vi "Main v0.2.vi"() -> ()   [LabVIEW 2017]
doc: "This template is for the Queued Message Handler design pattern.\n\nThe Event Handling Loop generates messages based on user interface actions.\n\nThe Message Handling Loop processes messages generated by the Event Handling Loop, or by other messages. The messages are string values, so new messages can be added easily to the Message Cases case structure in the Message Handling Loop. Each message cluster can also provide an optional value for Message Data, which is a variant that can be converted to whatever message-specific data is required."
uses:
  Controls/Main Tabs.ctl
  Controls/Auto.ctl
  RT/Controls/Auto Delays.ctl
  RT/Controls/Auto Times.ctl
  Controls/UI Data.ctl
  support/Message Queue/Enqueue Message (Single).vi
  <vilib>/Utility/error.llb/Error Cluster From Error Code.vi
  <vilib>/ErrorRing/Error Ring.xnode
  support/Message Queue/Message Queue.lvlib
  support/User Event - Stop/User Event - Stop.lvlib
panel:
  out "Date-Time":string caption="Dip-Tube Assembly Automation (HMI) v0.2"
  out "Main Tab":T1
  in  "Autocycle":T2
  in  "Manual":bool
  in  "Parameters":bool
  in  "Maintenance":bool
  in  "Save Para":bool
  in  "Home Para":bool
  in  "ParaTab":T3(tab)
  in  "StopperRearDelay":dbl format="%#.2f"
  in  "StopperFrontDelay":dbl format="%#.2f"
  in  "MaxAlarms":dbl caption="Max Alarms in 1 Minute" format="%#.2f"
  in  "MaxConsecutive":dbl caption="Max Consecutive Alarms" format="%#.2f"
  in  "Gate Close Delay":dbl format="%#.2f"
  in  "Gate Open Delay":dbl format="%#.2f"
  in  "BF Off Delay":dbl format="%#.2f"
  in  "BF On Delay":dbl format="%#.2f"
  in  "DelayAfterReject":dbl format="%#.2f"
  in  "MeasurementTime":dbl format="%#.2f"
  in  "DelayAfterMesFront":dbl format="%#.2f"
  in  "DelayAfterCut":dbl format="%#.2f"
  in  "DelayAfterCutClamp":dbl format="%#.2f"
  in  "DelayAfterInsClamp":dbl format="%#.2f"
  in  "DelayToClose":dbl format="%#.2f"
  in  "DelayToOpen":dbl format="%#.2f"
  in  "DelayAfterInsertion":dbl format="%#.2f"
  in  "DelayBeforeInsertion":dbl format="%#.2f"
  in  "AgitatorUpTime":dbl format="%#.2f"
  in  "AgitatorDownTime":dbl format="%#.2f"
  in  "Enable Index?":bool
  in  "Enable PF?":bool
  in  "Auto Delays":T4={"Agitator Delays"=[1000], "TF Delays"=[1000], "Insertion Delays"=[1000, 1000], "Cutting Delays"=[1000, 1000], "PF Delays"=[1000]}
  in  "Enable Cutting?":bool
  in  "Enable Insertion?":bool
  in  "Run Manual":bool
  in  "Enable TF?":bool
  in  "Home Manual":bool
  out "Status":T6
  in  "All IO":bool
  in  "Stats":bool
  in  "Home AC":bool
  out "Status":string
  out "Count":dbl format="%06.0f"
  out "Count 3":dbl caption="Cycle Time" format="%0.2f"
  out "Count 2":dbl caption="Rejects" format="%06.0f"
  in  "Statuses":string[][](table)
  in  "Exit":bool
  # "Vision Harmony Dip-Tube Assembly Automation"
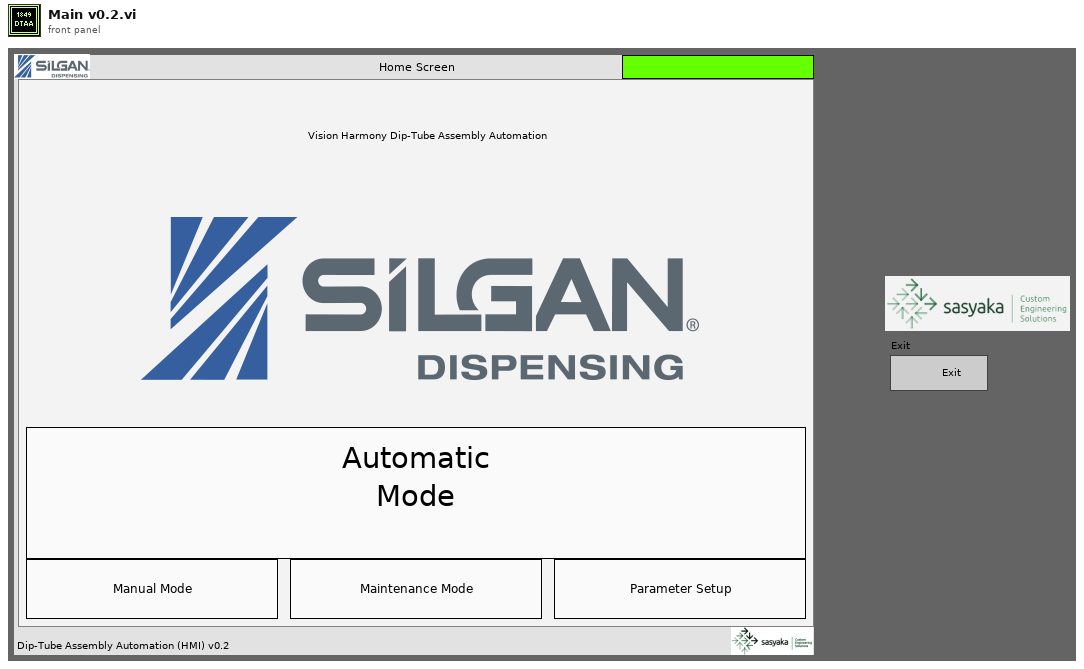
[diagram p1: front panel]
types:
  T1 = typedef "Main Tabs.ctl" = enum32{"Home Screen", "Parameter Setup", "Manual Mode", "Autocycle"}
  T2 = typedef "Auto.ctl" = bool
  T3 = enum32{"General & Indexing", "Bowl Feeder & Pump Conveyor", "Cutting, Measurement & Rejection", "Tube Feeder & Insertion"}
  T4 = typedef "Auto Delays.ctl" = cluster{"Agitator Delays":u32[], "TF Delays":u32[], "Insertion Delays":u32[], "Cutting Delays":u32[], "PF Delays":u32[]}
  T5 = typedef "Auto Times.ctl" = cluster{"Index Time":u32, "TF Time":u32, "Insertion Time":u32, "Cutting Time":u32, "PF Time":u32}
  T6 = cluster{"Auto Times":T5, "error out":errorcluster}
  T7 = typedef "UI Data.ctl" = cluster{"Main Tab":refnum<vi>}
  T8 = typedef "Message Queue.lvlib/All Message Queues.ctl" = cluster{"UI":refnum<queue>}
  T9 = enum8{"Enabled", "Disabled", "Disabled and Grayed Out"}
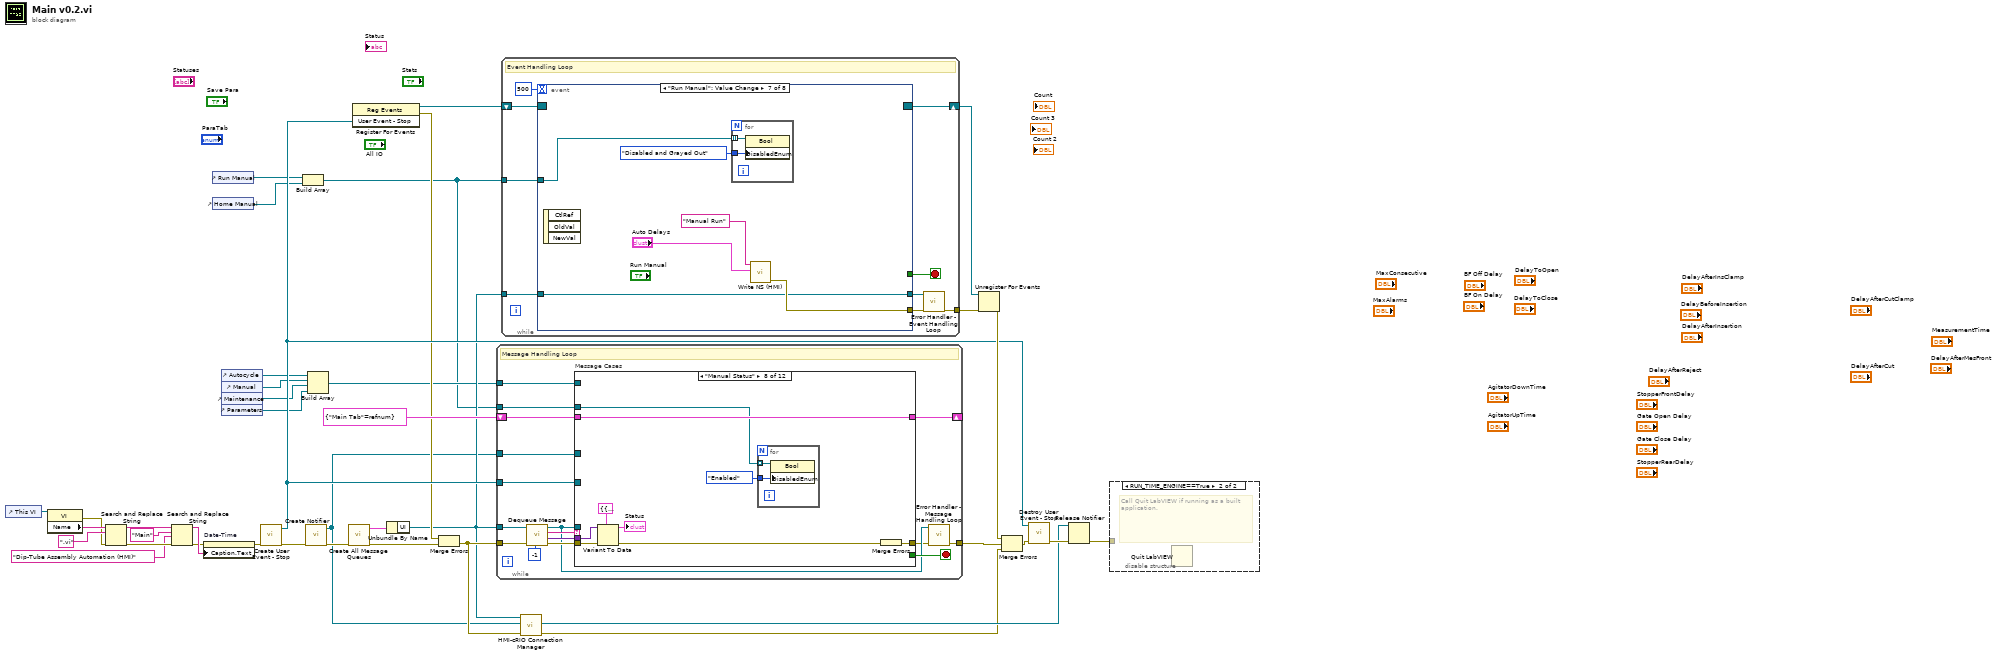
[diagram p0: block diagram]
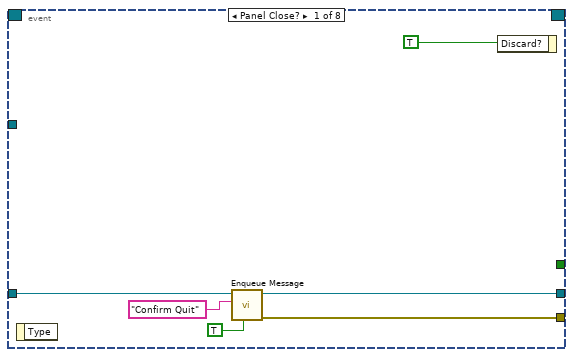
[diagram p2: hidden frame]
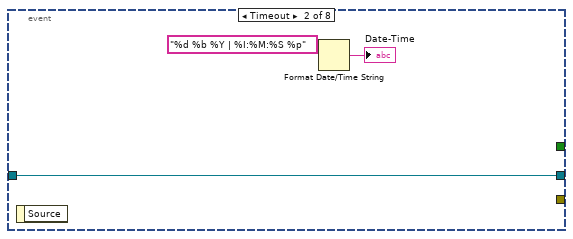
[diagram p3: hidden frame]
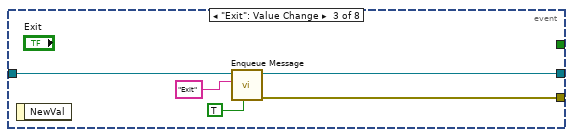
[diagram p4: hidden frame]
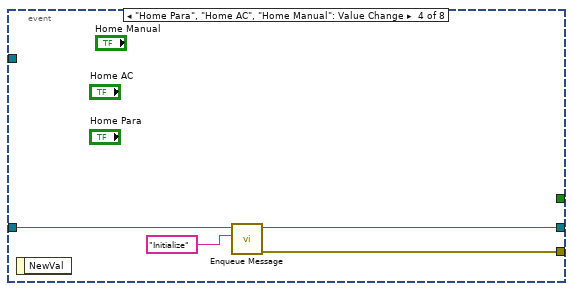
[diagram p5: hidden frame]
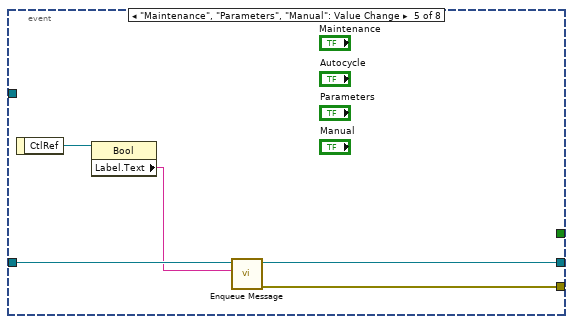
[diagram p6: hidden frame]
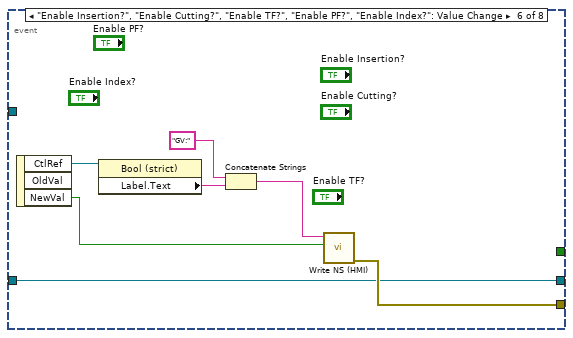
[diagram p7: hidden frame]
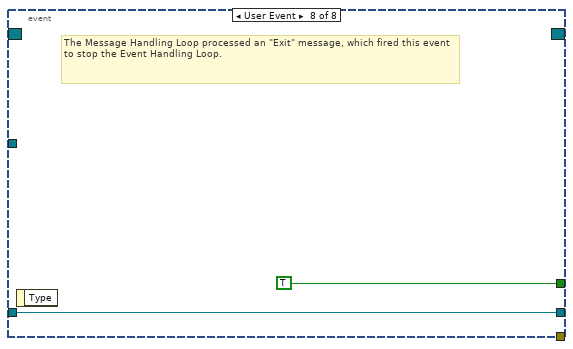
[diagram p8: hidden frame]
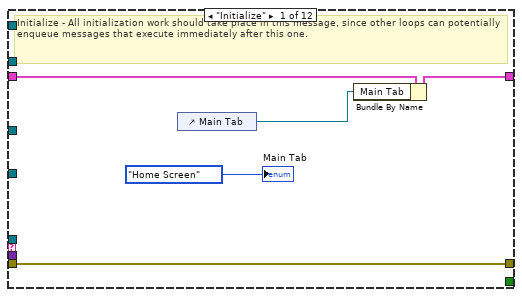
[diagram p9: hidden frame]
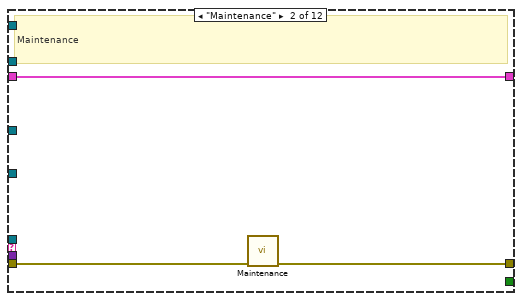
[diagram p10: hidden frame]
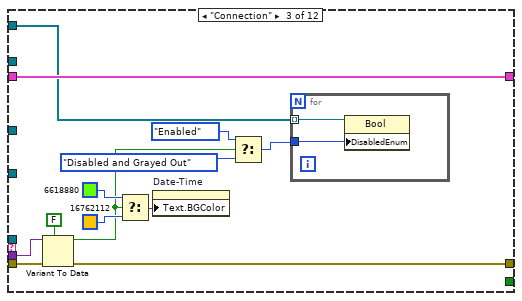
[diagram p11: hidden frame]
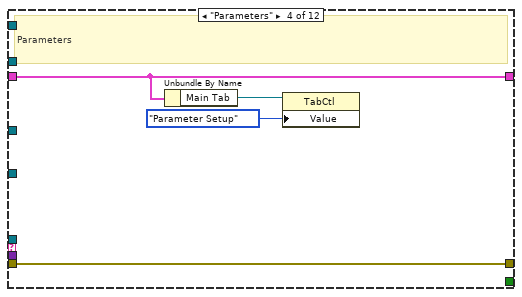
[diagram p12: hidden frame]
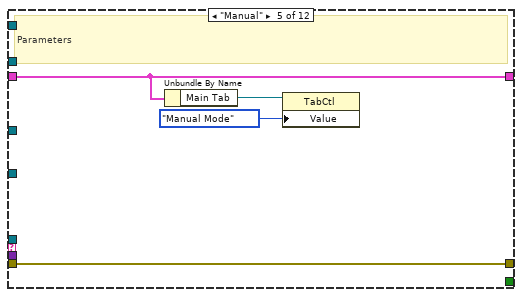
[diagram p13: hidden frame]
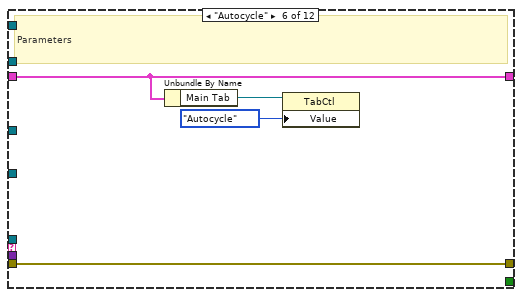
[diagram p14: hidden frame]
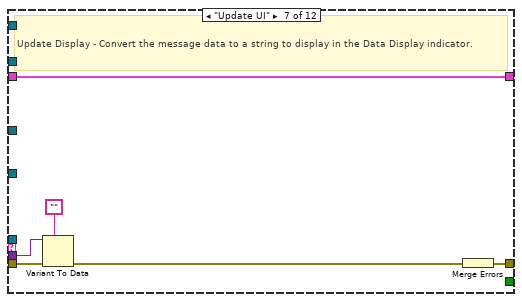
[diagram p15: hidden frame]
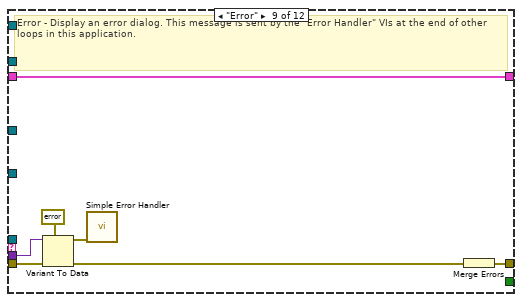
[diagram p16: hidden frame]
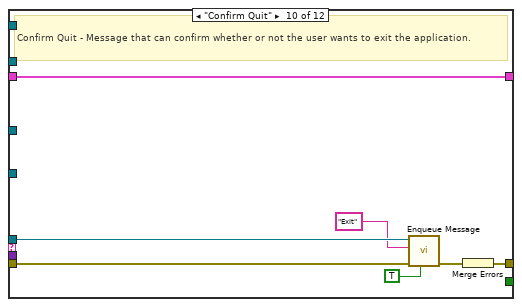
[diagram p17: hidden frame]
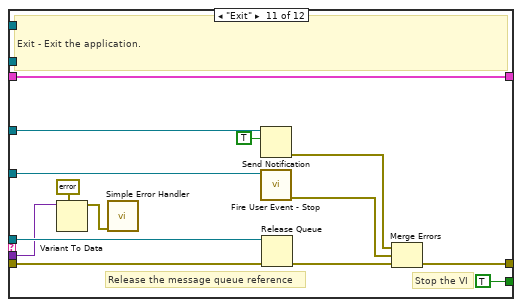
[diagram p18: hidden frame]
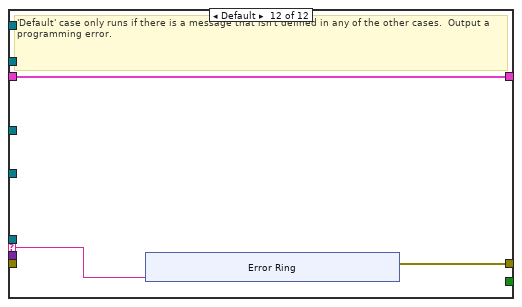
[diagram p19: hidden frame]
diagram:
  n1 = control-ref of="This VI"() -> (w8:refnum<vi>)
  n2 = property class="VI"(reference=w8) -> (error out=w7:errorcluster, "Name"=w14:string)  [unwired: 1 in, 1 out]
  n3 = Search and Replace String(input string=w14, search string=".vi", error in=w7) -> (result string=w12:string, error out=w11:errorcluster)  [unwired: 5 in, 2 out]
  n4 = Search and Replace String(input string=w12, search string="Main", replace string="Dip-Tube Assembly Automation (HMI)" ("replace string (\"\")"), error in=w11) -> (result string=w6:string, error out=w5:errorcluster)  [unwired: 4 in, 2 out]
  n5 = property on="Date-Time" class="Str"(error in=w5, "Caption.Text"=w6) -> (error out=w4:errorcluster)  [unwired: 1 in, 1 out]
  n6 = control-ref of="Run Manual"() -> (w3:refnum<vi>)
  n7 = control-ref of="Home Manual"() -> (w2:refnum<vi>)
  n8 = control-ref of="Autocycle"() -> (w19:refnum<vi>)
  n9 = control-ref of="Manual"() -> (w18:refnum<vi>)
  n10 = control-ref of="Maintenance"() -> (w17:refnum<vi>)
  n11 = control-ref of="Parameters"() -> (w16:refnum<vi>)
  n12 = call "Create User Event - Stop.vi"("error in (no error)"=w4) -> ("error out"=w26:errorcluster, "User Event - Stop"=w30:refnum<user-event>)  [unwired: 9 in]
  n13 = Build Array(w3, w2) -> (w1:refnum<vi>[])
  n14 = call "Create Notifier.vi"("error in (no error)"=w26) -> ("error out"=w25:errorcluster, "notifier out"=w20:refnum<notifier>)  [unwired: 9 in]
  n15 = Build Array(w19, w18, w17, w16) -> (w15:refnum<vi>[])
  n16 = call "Create All Message Queues.vi"("error in (no error)"=w25) -> ("error out"=w39:errorcluster, "Message Queues out"=w38:T8)  [unwired: 9 in]
  n17 = register-events(w30) -> (reference out=w31:refnum<event-registration>, error out=w29:errorcluster)  [unwired: 2 in]
  n18 = Unbundle By Name(w38) -> ("UI"=w27:refnum<queue>)
  n19 = Merge Errors(w29, w39) -> (w28:errorcluster)
  n20 = while {
    tunnel: w27 -> [w47]
    shift-right: [w54] -> _
    shift-left: T7 {"Main Tab"=refnum} ("Data Cluster") -> [w55]
    tunnel: w30 -> [w52]
    tunnel: w28 -> [w51]
    tunnel: [w45] -> w37
    tunnel: w20 -> [w42]
    tunnel: w15 -> [w41]
    tunnel: w1 -> [w40]
    stop <- w53 stop-if-true
    # "Message Handling Loop"
    n21 = call "Dequeue Message.vi"("timeout"=-1, "error in (no error)"=w51, "Message Queue"=w47) -> ("error out"=w50:errorcluster, "Message Data"=w48:variant, "Message"=w49:string, "dup Message Queue"=w46:refnum<queue>)  [unwired: 5 in]
    n22 = case "Message Cases" shown="\"Manual Status\"" w49 {
      selector: w49 -> [_ _ _ _ _ _ _ _ _ _ _ w136]
      tunnel: w46 -> [_ _ _ _ _ _ _ _ _ w117 w135 _]
      tunnel: w50 -> [w60 w62 w74 w82 w86 w90 w94 w103 w114 w121 w128 _]
      tunnel: [w60 w61 w73 w82 w86 w90 w95 w104 w108 w119 w131 w137] -> w44
      tunnel: w55 -> [w59 w63 w76 w81 w85 w89 w96 w105 w113 w120 w134 w138]
      tunnel: [w58 w63 w76 w81 w85 w89 w96 w105 w113 w120 w134 w138] -> w54
      tunnel: [_ _ _ _ _ _ _ _ _ _ TRUE _] -> w53
      tunnel: w48 -> [_ _ w72 _ _ _ w93 w102 w112 _ w125 _]
      tunnel: w52 -> [_ _ _ _ _ _ _ _ _ _ w130 _]
      tunnel: w42 -> [_ _ _ _ _ _ _ _ _ _ w124 _]
      tunnel: w41 -> [_ _ w68 _ _ _ _ _ _ _ _ _]
      tunnel: w40 -> [_ _ _ _ _ _ _ w97 _ _ _ _]
      frame "Initialize" {
        # "Initialize - All initialization work should take place in this message, since other loops can potentially enqueue messages that execute immediately after this one."
        n23 = control-ref of="Main Tab"() -> (w57:refnum<vi>)
        n24 = Bundle By Name(cluster=w59, "Main Tab"=w57) -> (w58:T7)
        "Main Tab" <- Main_Tabs."Home Screen" ("Main Tab")
      }
      frame "Maintenance" {
        # "Maintenance"
        n25 = call "Maintenance.vi"("Error In"=w62) -> ("Error out"=w61:errorcluster)  [unwired: 10 in]
      }
      frame "Connection" {
        n26 = Variant To Data(error in=w74, type=FALSE, Variant=w72) -> (data=w67:bool, error out=w73:errorcluster)
        n27 = Select(t=u32 6618880 ("Text.Text Colors:BG Color"), s=w67, f=u32 16762112 ("Text.Text Colors:BG Color")) -> (s? t:f=w69:u32)
        n28 = property on="Date-Time" class="Str"("Text.BGColor"=w69) -> ()  [unwired: 2 in, 2 out]
        n29 = Select(t=T9."Enabled" ("Disabled"), s=w67, f=T9."Disabled and Grayed Out") -> (s? t:f=w65:T9)
        n30 = for {
          tunnel: w68 -> [w78] mode=indexing
          tunnel: w65 -> [w77]
          n31 = property class="Bool"(reference=w78, "DisabledEnum"=w77) -> ()  [unwired: 1 in, 2 out]
        }
      }
      frame "Parameters" {
        # "Parameters"
        n32 = Unbundle By Name(w81) -> ("Main Tab"=w80:refnum<vi>)
        n33 = property class="TabCtl"(reference=w80, "Value"=Main_Tabs."Parameter Setup" ("Main Tab")) -> ()  [unwired: 1 in, 2 out]
      }
      frame "Manual" {
        # "Parameters"
        n34 = Unbundle By Name(w85) -> ("Main Tab"=w84:refnum<vi>)
        n35 = property class="TabCtl"(reference=w84, "Value"=Main_Tabs."Manual Mode" ("Main Tab")) -> ()  [unwired: 1 in, 2 out]
      }
      frame "Autocycle" {
        # "Parameters"
        n36 = Unbundle By Name(w89) -> ("Main Tab"=w88:refnum<vi>)
        n37 = property class="TabCtl"(reference=w88, "Value"=Main_Tabs."Autocycle" ("Main Tab")) -> ()  [unwired: 1 in, 2 out]
      }
      frame "Update UI" {
        # "Update Display - Convert the message data to a string to display in the Data Display indicator."
        n38 = Variant To Data(error in=w94, type="", Variant=w93) -> (error out=w91:errorcluster)  [unwired: 1 out]
        n39 = Merge Errors(w91) -> (w95:errorcluster)
      }
      frame "Manual Status" {
        n40 = Variant To Data(error in=w103, type=T6 {"Auto Times"={"Index Time"=0, "TF Time"=0, "Insertion Time"=0, "Cutting Time"=0, "PF Time"=0}, "error out"={"status"=FALSE, "code"=0, "source"=""}} ("cluster"), Variant=w102) -> (data=→"Status":T6, error out=w101:errorcluster)
        n41 = for {
          tunnel: w97 -> [w107] mode=indexing
          tunnel: T9."Enabled" ("Disabled") -> [w106]
          n42 = property class="Bool"(reference=w107, "DisabledEnum"=w106) -> ()  [unwired: 1 in, 2 out]
        }
        n43 = Merge Errors(w101) -> (w104:errorcluster)
      }
      frame "Error" {
        # "Error - Display an error dialog. This message is sent by the \"Error Handler\" VIs at the end of other loops in this application."
        n44 = Variant To Data(error in=w114, type=errorcluster {"status"=FALSE, "code"=0, "source"=""} ("error constant"), Variant=w112) -> (data=w110:errorcluster, error out=w109:errorcluster)
        n45 = call <vilib>:"Simple Error Handler.vi"("error in (no error)"=w110) -> ()  [unwired: 4 in, 5 out]
        n46 = Merge Errors(w109) -> (w108:errorcluster)
      }
      frame "Confirm Quit" {
        # "Confirm Quit - Message that can confirm whether or not the user wants to exit the application."
        n47 = call-poly "Enqueue Message.vi"("Priority Message? (F)"=TRUE, "error in (no error)"=w121, "Message"="Exit", "Message Queue"=w117) -> ("error out"=w118:errorcluster)  [unwired: 6 in, 1 out]
        n48 = Merge Errors(w118) -> (w119:errorcluster)
      }
      frame "Exit" {
        # "Stop the VI"
        # "Release the message queue reference"
        # "Exit - Exit the application."
        n49 = Variant To Data(type=errorcluster {"status"=FALSE, "code"=0, "source"=""} ("error constant"), Variant=w125) -> (data=w126:errorcluster)  [unwired: 1 in, 1 out]
        n50 = call <vilib>:"Simple Error Handler.vi"("error in (no error)"=w126) -> ()  [unwired: 4 in, 5 out]
        n51 = Send Notification(notification=TRUE, notifier=w124) -> (error out=w122:errorcluster)  [unwired: 1 in, 1 out]
        n52 = call "Fire User Event - Stop.vi"("User Event - Stop"=w130) -> ("error out"=w129:errorcluster)  [unwired: 10 in]
        n53 = Release Queue(queue=w135, error in (no error)=w128) -> (error out=w132:errorcluster)  [unwired: 1 in, 2 out]
        n54 = Merge Errors(w122, w129, w132) -> (w131:errorcluster)
      }
      frame Default {
        # "'Default' case only runs if there is a message that isn't defined in any of the other cases.  Output a programming error."
        n55 = xnode "Error Ring"("parameter 0"=w136) -> ("error out"=w137:errorcluster)
      }
    }
    n56 = call "Error Handler - Message Handling Loop.vi"("error in (no error)"=w44, "Message Queue"=w46) -> ("dup error in"=w45:errorcluster)  [unwired: 8 in, 1 out]
  }
  n57 = while {
    tunnel: w27 -> [w154]
    shift-right: [w152] -> w34
    shift-left: w31 -> [w153]
    tunnel: [w148] -> w32
    tunnel: w1 -> [w146]
    stop <- w150 stop-if-true
    # "Event Handling Loop"
    n58 = event shown="[6] \"Run Manual\": Value Change" {
      selector: w153 -> [_ _ _ _ _ _ _ _]
      dyn-events: [_ _ _ _ _ _ _ _] -> w152
      timeout: 500 -> [_ _ _ _ _ _ _ _]
      tunnel: [_ _ _ _ _ _ _ TRUE ("Discard?")] -> w150
      tunnel: w154 -> [w159 w163 w168 w172 w177 w182 w189 w194]
      tunnel: [w158 _ w167 w171 w176 w183 w190 _] -> w151
      tunnel: [w157 w163 w166 w170 w175 w182 w189 w194] -> w149
      tunnel: w146 -> [_ _ _ _ _ _ w186 _]
      event Panel Close? {
        n59 = event-data() -> ()  [unwired: 1 in, 1 out]
        n60 = call-poly "Enqueue Message.vi"("Priority Message? (F)"=TRUE, "Message"="Confirm Quit", "Message Queue"=w159) -> ("error out"=w158:errorcluster, "dup Message Queue"=w157:refnum<queue>)  [unwired: 7 in]
        n61 = event-data("Discard?"=TRUE) -> ()  [unwired: 1 in, 1 out]
      }
      event Timeout {
        n62 = event-data() -> ()  [unwired: 1 in, 1 out]
        n63 = Format Date/Time String(time format string (%c)="%d %b %Y | %I:%M:%S %p") -> (date/time string=→"Date-Time":string)  [unwired: 2 in]
      }
      event "Exit": Value Change {
        n64 = event-data() -> ()  [unwired: 1 in, 1 out]
        n65 = call-poly "Enqueue Message.vi"("Priority Message? (F)"=TRUE, "Message"="Exit", "Message Queue"=w168) -> ("error out"=w167:errorcluster, "dup Message Queue"=w166:refnum<queue>)  [unwired: 7 in]
      }
      event "Home Para", "Home AC", "Home Manual": Value Change {
        n66 = event-data() -> ()  [unwired: 1 in, 1 out]
        n67 = call-poly "Enqueue Message.vi"("Message"="Initialize", "Message Queue"=w172) -> ("error out"=w171:errorcluster, "dup Message Queue"=w170:refnum<queue>)  [unwired: 8 in]
      }
      event "Maintenance", "Parameters", "Manual": Value Change {
        n68 = event-data() -> ("CtlRef"=w174:refnum<vi>)  [unwired: 1 in]
        n69 = property class="Bool"(reference=w174) -> ("Label.Text"=w173:string)  [unwired: 1 in, 2 out]
        n70 = call-poly "Enqueue Message.vi"("Message"=w173, "Message Queue"=w177) -> ("error out"=w176:errorcluster, "dup Message Queue"=w175:refnum<queue>)  [unwired: 8 in]
      }
      event "Enable Insertion?", "Enable Cutting?", "Enable TF?", "Enable PF?", "Enable Index?": Value Change {
        n71 = event-data() -> ("CtlRef"=w184:refnum<vi>, "NewVal"=w178:bool)  [unwired: 1 in, 1 out]
        n72 = property class="Bool (strict)"(reference=w184) -> ("Label.Text"=w181:string)  [unwired: 1 in, 2 out]
        n73 = Concatenate Strings("GV:" ("string"), w181) -> (w179:string)
        n74 = call "Write NS (HMI).vi"("Message Data"=w178, "Message"=w179) -> ("error out"=w183:errorcluster)  [unwired: 9 in]
      }
      event "Run Manual": Value Change {
        n75 = event-data() -> ()  [unwired: 1 in, 3 out]
        n76 = for {
          tunnel: w186 -> [w192] mode=indexing
          tunnel: T9."Disabled and Grayed Out" ("Disabled") -> [w191]
          n77 = property class="Bool"(reference=w192, "DisabledEnum"=w191) -> ()  [unwired: 1 in, 2 out]
        }
        n78 = call "Write NS (HMI).vi"("Message Data"="Auto Delays", "Message"="Manual Run") -> ("error out"=w190:errorcluster)  [unwired: 9 in]
      }
      event User Event {
        # "The Message Handling Loop processed an \"Exit\" message, which fired this event to stop the Event Handling Loop."
        n79 = event-data() -> ()  [unwired: 1 in, 1 out]
      }
    }
    n80 = call "Error Handler - Event Handling Loop.vi"("error in (no error)"=w151, "Message Queue"=w149) -> ("dup error in"=w148:errorcluster)  [unwired: 8 in, 1 out]
  }
  n81 = call "HMI-cRIO Connection Manager.vi"("error in"=w28, "notifier in"=w20, "Queue in"=w27) -> ("error out"=w21:errorcluster, "Notifier out"=w22:refnum<notifier>)  [unwired: 7 in]
  n82 = Unregister For Events(event registration refnum=w34, error in=w32) -> (error out=w35:errorcluster)
  n83 = Merge Errors(w35, w37, w21) -> (w36:errorcluster)
  n84 = call "Destroy User Event - Stop.vi"("error in (no error)"=w36, "User Event - Stop"=w30) -> ("error out"=w24:errorcluster)  [unwired: 9 in]
  n85 = Release Notifier(notifier=w22, error in (no error)=w24) -> (error out=w23:errorcluster)  [unwired: 1 in, 2 out]
  n86 = disable-structure shown="RUN_TIME_ENGINE==True" {
    disable-tunnel: w23 -> [_ _]
    frame condition #0 (active) {
    }
    frame condition #1 {
      # "Call Quit LabVIEW if running as a built application."
      n87 = Quit LabVIEW() -> ()  [unwired: 1 in]
    }
  }
